vi "溢出.vi"() -> ()   [LabVIEW 2020]
panel:
  in  "数值 3":i16
  in  "数值 2":i16
  out "数值":i16
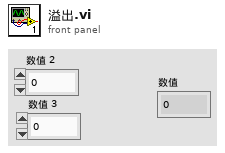
[diagram p1: front panel]
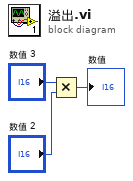
[diagram p0: block diagram]
diagram:
  n1 = Multiply(x="数值 3", y="数值 2") -> (x*y=→"数值":i16)
